vi "浮点转字节数组.vi"(2 "输入":dbl) -> (1 "数组，高字节在前":u8[](array[numeric]) format="0x%x", 5 "高字节":u16, 6 "次高":u8, 7 "次低":u8, 8 "低字节":u8)   [LabVIEW 2017]
panel:
  # "放大100倍的数"
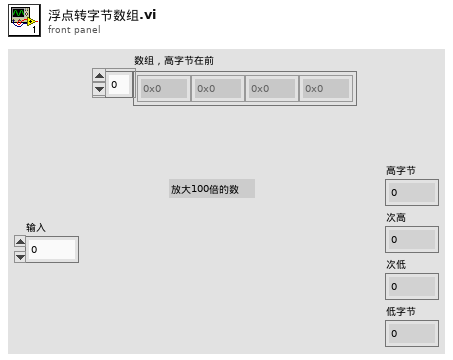
[diagram p1: front panel]
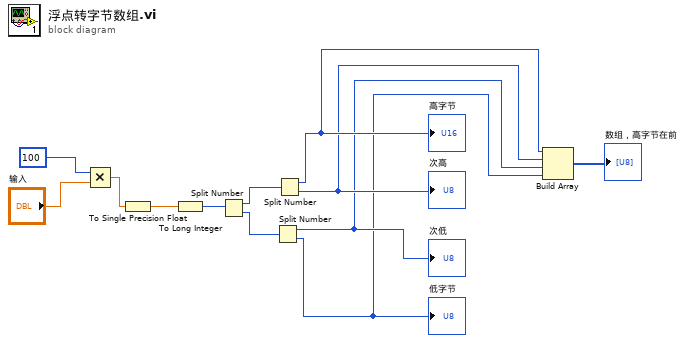
[diagram p0: block diagram]
diagram:
  n1 = Multiply(x=100, y="输入") -> (x*y=w1:dbl)
  n2 = To Single Precision Float(number=w1) -> (single precision float=w10:sgl)
  n3 = To Long Integer(number=w10) -> (32bit integer=w9:i32)
  n4 = Split Number(x=w9) -> (hi(x)=w12:u16, lo(x)=w11:u16)
  n5 = Split Number(x=w11) -> (hi(x)=w6:u8, lo(x)=w5:u8)
  "次低" <- w6
  "低字节" <- w5
  n6 = Split Number(x=w12) -> (hi(x)=w8:u8, lo(x)=w7:u8)
  "高字节" <- w8
  "次高" <- w7
  n7 = Build Array(w8, w7, w6, w5) -> (→"数组，高字节在前":u8[])
